vi "ErrorHandlerSubVI.vi"(2 "Errors":errorcluster[](array[cluster]), 3 "queue in":refnum<queue>, 4 "Conections In":T1 {"VISAs"."Stop bit" items=["1.0"=10, "1.5"=15, "2.0"=20]; "VISAs"."Parity" items=["No parity", "Odd parity", "Even parity", "Mark parity", "Space parity"]}) -> (0 "Status":string[](array[string]), 1 "queue out":refnum<queue>)   [LabVIEW 2016]
doc: "Filters all the errors and returns an array of <b>status</b>"
panel:
  in  "VISA resource name":refnum<visa-resource-name>
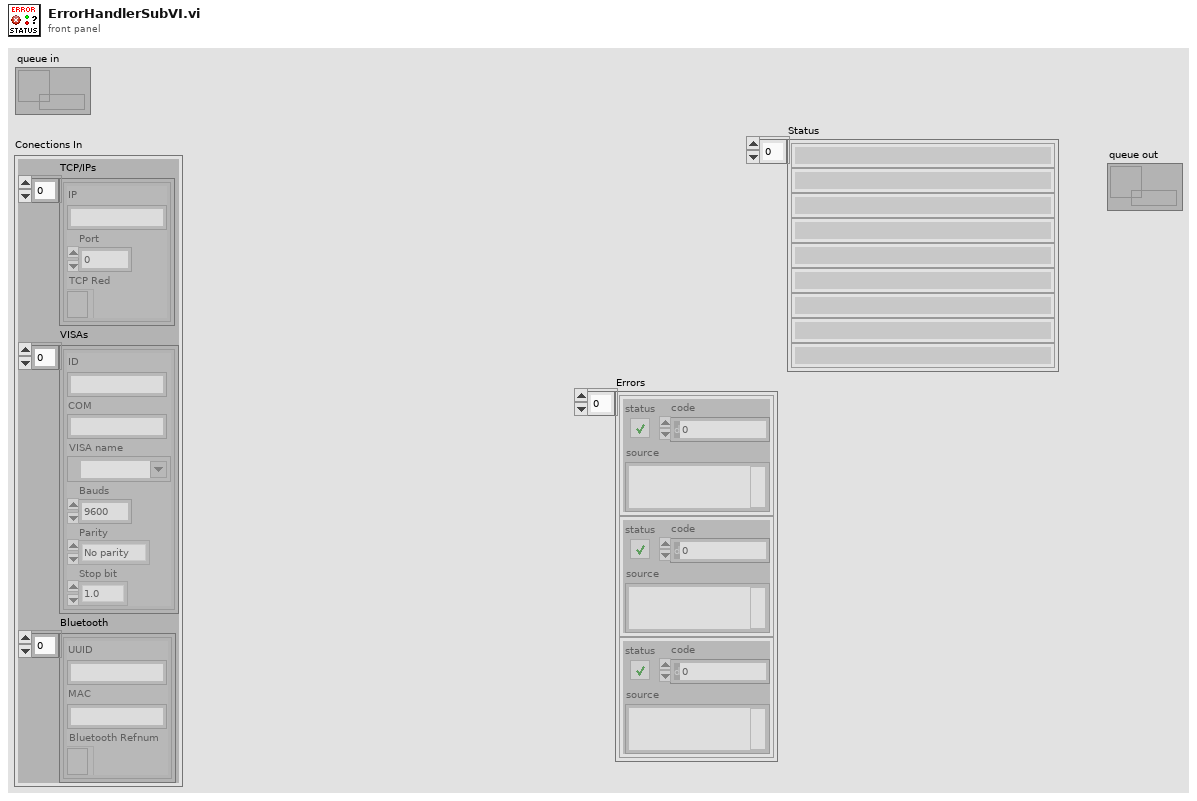
[diagram p1: front panel]
types:
  T1 = cluster{"TCP/IPs":cluster{"IP":string, "Port":u16, "TCP Red":refnum<k5>}[], "VISAs":cluster{"ID":string, "COM":string, "VISA name":refnum<visa-resource-name>, "Bauds":dbl, "Parity":u16, "Stop bit":u16}[], "Bluetooth":cluster{"UUID":string, "MAC":string, "Bluetooth Refnum":refnum<k31>}[]}
  T2 = cluster{"ID":string, "COM":string, "VISA name":refnum<visa-resource-name>, "Bauds":dbl, "Parity":u16, "Stop bit":u16}[]
  T3 = cluster{"ID":string, "COM":string, "VISA name":refnum<visa-resource-name>, "Bauds":dbl, "Parity":u16, "Stop bit":u16}
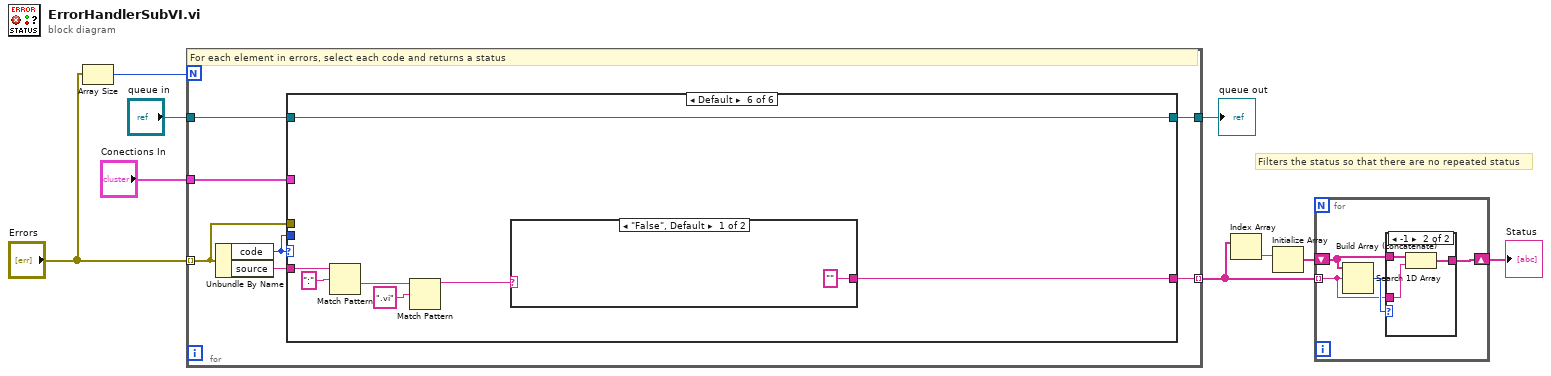
[diagram p0: block diagram]
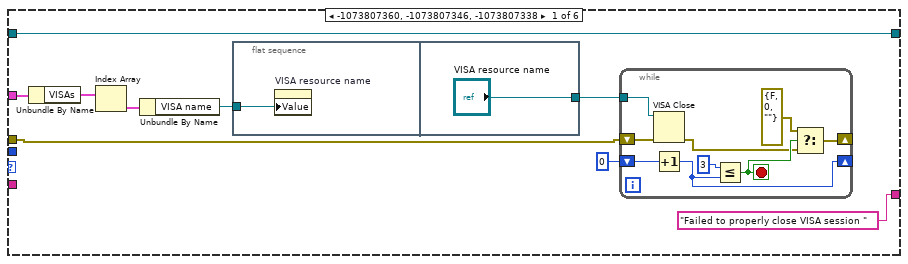
[diagram p3: hidden frame]
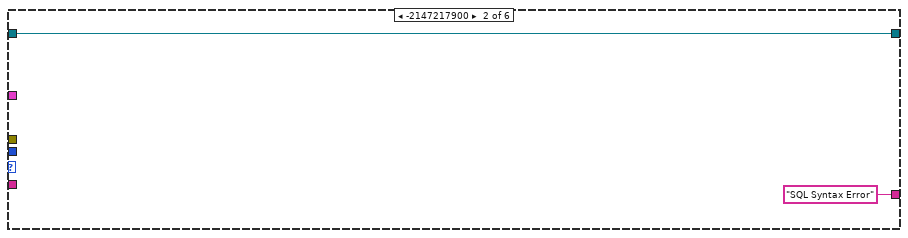
[diagram p4: hidden frame]
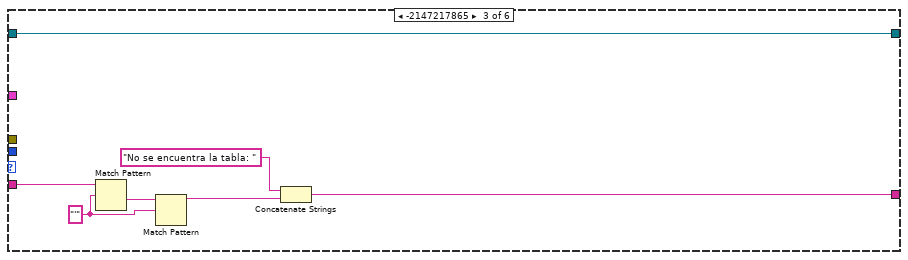
[diagram p5: hidden frame]
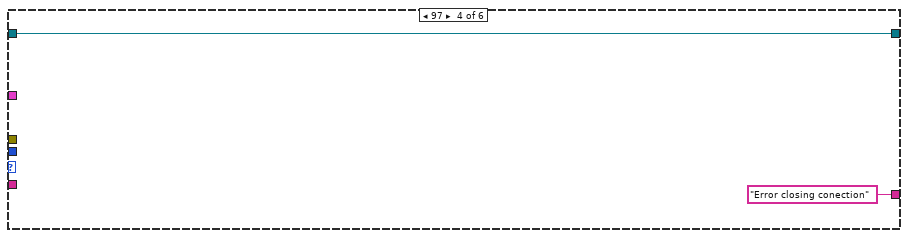
[diagram p6: hidden frame]
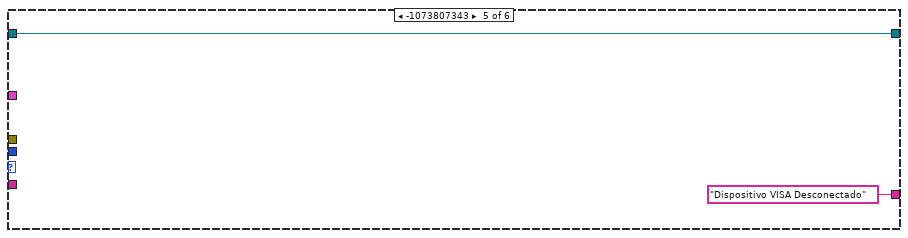
[diagram p7: hidden frame]
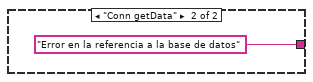
[diagram p8: hidden frame]
diagram:
  # "Filters the status so that there are no repeated status"
  n1 = Array Size(array="Errors") -> (size(s)=w9:i32)
  n2 = for {
    N: w9 -> [_]
    tunnel: "Errors" -> [w10] mode=indexing
    tunnel: "Conections In" -> [w16]
    tunnel: "queue in" -> [w15]
    tunnel: [w12] -> w2 mode=indexing
    tunnel: [w13] -> w7
    # "For each element in errors, select each code and returns a status"
    n3 = Unbundle By Name(w10) -> ("code"=w11:i32, "source"=w14:string)
    n4 = case shown="Default" w11 {
      tunnel: w14 -> [_ _ w42 _ _ w55]
      tunnel: w15 -> [w18 w37 w45 w47 w48 w56]
      tunnel: [w18 w37 w45 w47 w48 w56] -> w13
      tunnel: ["Failed to properly close VISA session " "SQL Syntax Error" w44 "Error closing conection" "Dispositivo VISA Desconectado" w50] -> w12
      tunnel: w16 -> [w24 _ _ _ _ _]
      tunnel: w11 -> [_ _ _ _ _ _]
      tunnel: w10 -> [w17 _ _ _ _ _]
      frame -1073807360, -1073807346, -1073807338 {
        n5 = Unbundle By Name(w24) -> ("VISAs"=w22:T2)
        n6 = Index Array(array=w22) -> (element=w23:T3)  [unwired: 1 in]
        n7 = Unbundle By Name(w23) -> ("VISA name"=w20:refnum<visa-resource-name>)
        n8 = flat-sequence {
          tunnel: w20 -> [w35]
          tunnel: ["VISA resource name"] -> w21
          frame #0 {
            n9 = property on="VISA resource name" class="VISAName"("Value"=w35) -> ()  [unwired: 2 in, 2 out]
          }
          frame #1 {
          }
        }
        n10 = while {
          tunnel: w21 -> [w34]
          shift-right: [w28] -> _
          shift-left: 0 -> [w30]
          shift-right: [w32] -> _
          shift-left: w17 -> [w33]
          stop <- w31 stop-if-true
          n11 = VISA Close(VISA resource name=w34, error in (no error)=w33) -> (error out=w27:errorcluster)
          n12 = Increment(x=w30) -> (x+1=w28:i32)
          n13 = Less Or Equal?(x=3, y=w28) -> (x <= y?=w31:bool)
          n14 = Select(t=errorcluster {"status"=FALSE, "code"=0, "source"=""} ("f"), s=w31, f=w27) -> (s? t:f=w32:errorcluster)
        }
      }
      frame -2147217900 {
      }
      frame -2147217865 {
        w40 = "'" ("search string/char (-)")
        n15 = Match Pattern(string=w42, regular expression=w40) -> (after substring=w41:string)  [unwired: 1 in, 3 out]
        n16 = Match Pattern(string=w41, regular expression=w40) -> (before substring=w39:string)  [unwired: 1 in, 3 out]
        n17 = Concatenate Strings("No se encuentra la tabla: ", w39) -> (w44:string)
      }
      frame 97 {
      }
      frame -1073807343 {
      }
      frame Default {
        n18 = Match Pattern(string=w55, regular expression=":") -> (after substring=w52:string)  [unwired: 1 in, 3 out]
        n19 = Match Pattern(string=w52, regular expression=".vi") -> (before substring=w51:string)  [unwired: 1 in, 3 out]
        n20 = case shown="\"False\", Default" w51 {
          tunnel: ["" "Error en la referencia a la base de datos"] -> w50
          frame "False", Default {
          }
          frame "Conn getData" {
          }
        }
      }
    }
  }
  "queue out" <- w7
  n21 = Index Array(array=w2) -> (element=w5:string)  [unwired: 1 in]
  n22 = Initialize Array(w5) -> (w6:string[])  [unwired: 1 in]
  n23 = for {
    tunnel: w2 -> [w61] mode=indexing
    shift-right: [w59] -> w4
    shift-left: w6 -> [w60]
    n24 = Search 1D Array(1D array=w60, element=w61) -> (index of element=w62:i32)  [unwired: 1 in]
    n25 = case shown="-1" w62 {
      tunnel: w61 -> [_ w66]
      tunnel: w60 -> [w63 w65]
      tunnel: [w63 w64] -> w59
      frame 0, Default {
      }
      frame -1 {
        n26 = Build Array (concatenate)(w65, w66) -> (w64:string[])
      }
    }
  }
  "Status" <- w4
